vi "VCS Get Position Regulator Feed Forward.vi"(0 "axis in":cluster{"keyHandle":u32, "nodeId":u16}={"keyHandle"=0, "nodeId"=1}, 11 "error in (no error)":errorcluster) -> (4 "axis out":cluster{"keyHandle":u32, "nodeId":u16}={"keyHandle"=0, "nodeId"=1}, 6 "feed forward":T1, 15 "error out":errorcluster)   [LabVIEW 2010]
doc: "<B>VCS_GetPositionRegulatorFeedForward</B> reads parameters for position regulation feed forward."
uses:
  Resources/EposCmd.dll
  Resources/EposCmd64.dll
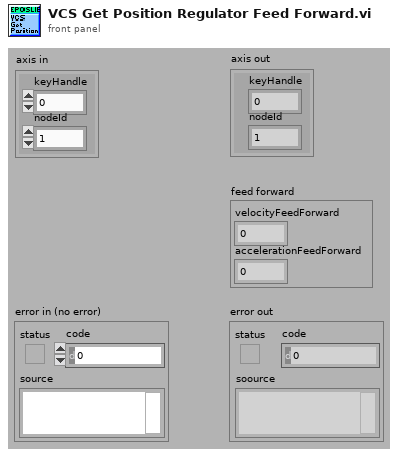
[diagram p1: front panel]
types:
  T1 = cluster{"velocityFeedForward":u16, "accelerationFeedForward":u16}
  T2 = cluster{"pVelocityFeedForward":u16, "pAccelerationFeedForward":u16}
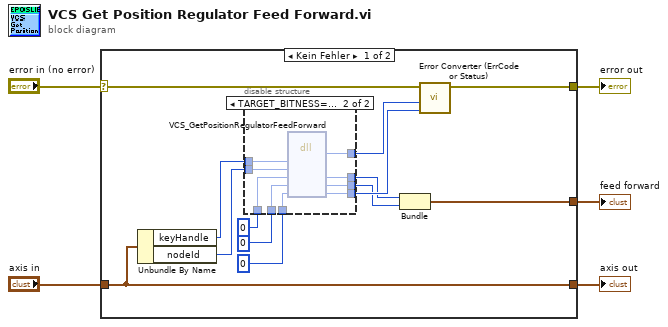
[diagram p0: block diagram]
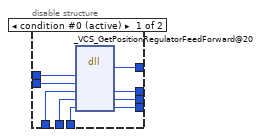
[diagram p2: hidden frame]
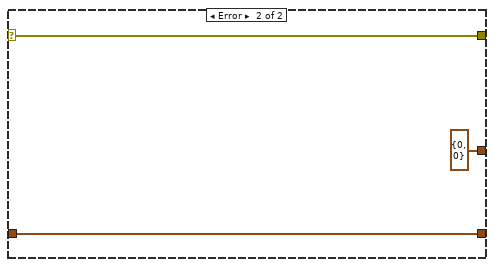
[diagram p3: hidden frame]
diagram:
  n1 = case shown="Kein Fehler" "error in (no error)" {
    selector: "error in (no error)" -> [w16 w38]
    tunnel: "axis in" -> [w18 w39]
    tunnel: [w18 w39] -> w4
    tunnel: [w17 w38] -> w3
    tunnel: [w6 T2 {"pVelocityFeedForward"=0, "pAccelerationFeedForward"=0}] -> w1
    frame No Error {
      n2 = Unbundle By Name(w18) -> ("keyHandle"=w14:u32, "nodeId"=w13:u16)
      n3 = disable-structure shown="TARGET_BITNESS==64" {
        disable-tunnel: u32 0 ("pErrorCode") -> [w27 w36]
        disable-tunnel: w14 -> [w26 w35]
        disable-tunnel: w13 -> [w25 w34]
        disable-tunnel: u16 0 ("pVelocityFeedForward") -> [w24 w33]
        disable-tunnel: u16 0 ("pAccelerationFeedForward") -> [w23 w32]
        disable-tunnel: [w22 w31] -> w10
        disable-tunnel: [w21 w30] -> w9
        disable-tunnel: [w20 w29] -> w8
        disable-tunnel: [w19 w28] -> w7
        frame condition #0 (active) {
          n4 = dll-call lib="C:/Sources/LabView/maxon EPOS/Resources/EposCmd.*" fn="_VCS_GetPositionRegulatorFeedForward@20"("KeyHandle"=w26, "NodeId"=w25, "pVelocityFeedForward"=w24, "pAccelerationFeedForward"=w23, "pErrorCode"=w27) -> (w21:i32, "pVelocityFeedForward"=w20:u16, "pAccelerationFeedForward"=w19:u16, "pErrorCode"=w22:u32)  [unwired: 5 in, 2 out]
        }
        frame condition #1 {
          n5 = dll-call lib="C:/setup/Resources/EposCmd64.dll" fn="VCS_GetPositionRegulatorFeedForward" ("EposCmd.dll:_VCS_GetPositionRegulatorFeedForward@20")("KeyHandle"=w35, "NodeId"=w34, "pVelocityFeedForward"=w33, "pAccelerationFeedForward"=w32, "pErrorCode"=w36) -> ("Rückgabetyp"=w30:i32, "pVelocityFeedForward"=w29:u16, "pAccelerationFeedForward"=w28:u16, "pErrorCode"=w31:u32)  [unwired: 5 in, 2 out]
        }
      }
      n6 = Bundle("pVelocityFeedForward"=w8, "pAccelerationFeedForward"=w7) -> (w6:T2)  [unwired: 1 in]
      n7 = call "Error Converter (ErrCode or Status).vi"("error code"=w10, "return type"=w9, "error in (no error)"=w16) -> ("error out"=w17:errorcluster)  [unwired: 7 in]
    }
    frame Error {
    }
  }
  "error out" <- w3
  "axis out" <- w4
  "feed forward" <- w1
